vi "Init Async State Vars.vi"(8 "Error in":errorcluster, 10 "Async Parameters":T4) -> (0 "Error out":errorcluster, 3 "Async State Vars":T1)   [LabVIEW 2015, in "Waveform-Processing-Custom-Device Engine.lvlib"]
uses:
  Waveform-Processing-Custom-Device Engine.lvlib
  Types/Async Parameters.ctl
  Types/Async FIFOs.ctl
  <vilib>/NI Veristand/Custom Device API/Waveform Data Reference.ctl
  Types/Async State Vars.ctl
  <vilib>/NI Veristand/Custom Device Waveform API/Single Waveform Read (DBL)/Single Waveform Read (DBL).lvclass
  <vilib>/NI Veristand/Custom Device Waveform API/Single Waveform Write (DBL)/Single Waveform Write (DBL).lvclass
  <vilib>/NI VeriStand/Custom Device API/Custom Device API.lvlib
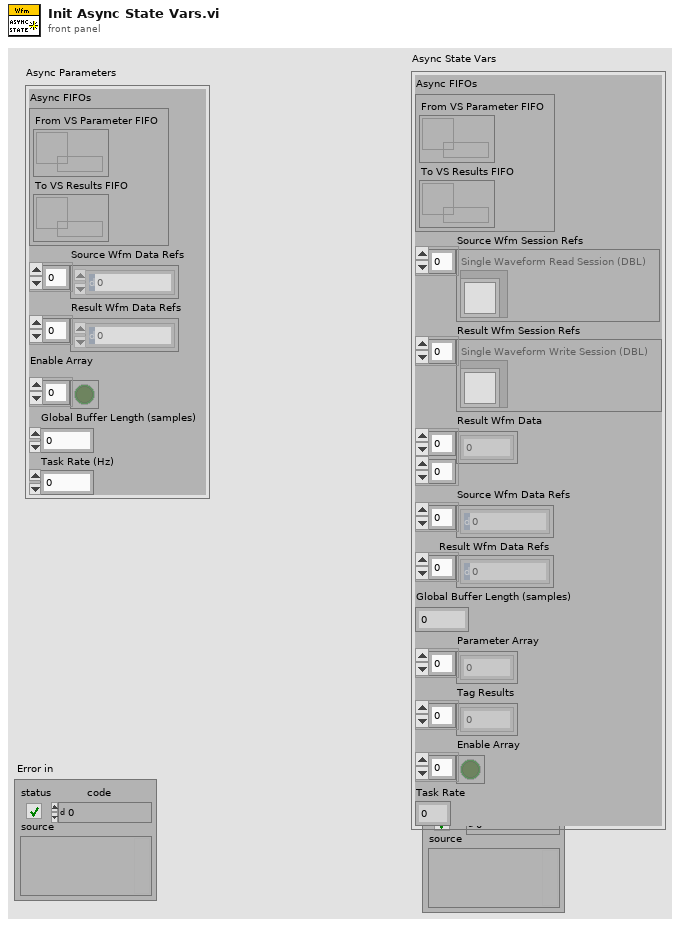
[diagram p1: front panel]
types:
  T1 = typedef "Waveform-Processing-Custom-Device Engine.lvlib/Async State Vars.ctl" = cluster{"Async FIFOs":T2, "Source Wfm Session Refs":refnum<class "Single Waveform Read (DBL).lvclass">[], "Result Wfm Session Refs":refnum<class "Single Waveform Write (DBL).lvclass">[], "Result Wfm Data":dbl[][], "Source Wfm Data Refs":T3[], "Result Wfm Data Refs":T3[], "Global Buffer Length (samples)":dbl, "Parameter Array":dbl[], "Tag Results":dbl[], "Enable Array":bool[], "Task Rate":dbl}
  T2 = typedef "Waveform-Processing-Custom-Device Engine.lvlib/Async FIFOs.ctl" = cluster{"From VS Parameter FIFO":refnum<k33>, "To VS Results FIFO":refnum<k33>}
  T3 = typedef "Custom Device API.lvlib/Waveform Data Reference.ctl" = i32
  T4 = typedef "Waveform-Processing-Custom-Device Engine.lvlib/Async Parameters.ctl" = cluster{"Async FIFOs":T2, "Source Wfm Data Refs":T3[], "Result Wfm Data Refs":T3[], "Enable Array":bool[], "Global Buffer Length (samples)":dbl, "Task Rate (Hz)":dbl}
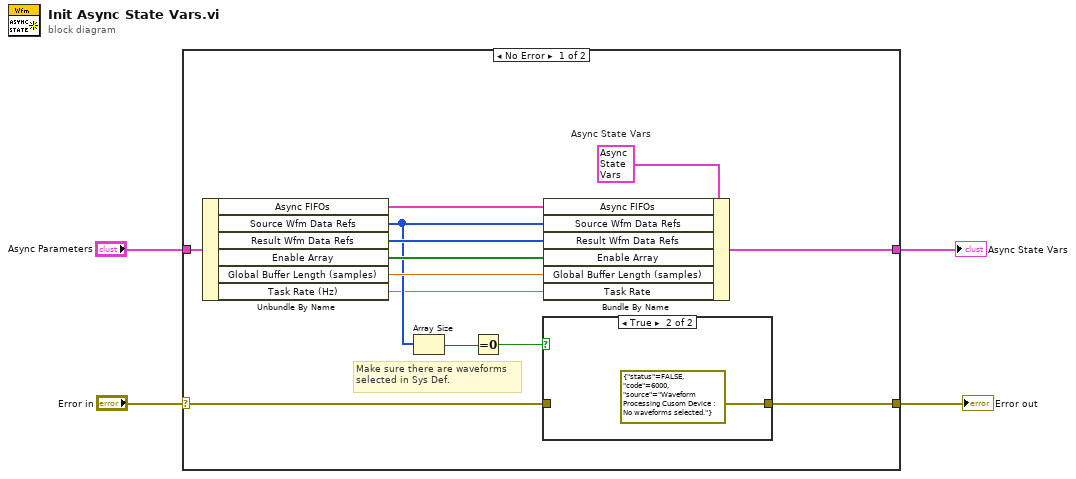
[diagram p0: block diagram]
diagram:
  n1 = case shown="No Error" "Error in" {
    selector: "Error in" -> [w7 w20]
    tunnel: [w6 w20] -> w3
    tunnel: "Async Parameters" -> [w17 _]
    tunnel: [w13 _] -> w1
    frame No Error {
      w16 = T1 {"Async FIFOs"={"From VS Parameter FIFO"=refnum, "To VS Results FIFO"=refnum}, "Source Wfm Session Refs"=[], "Result Wfm Session Refs"=[], "Result Wfm Data"=[], "Source Wfm Data Refs"=[], "Result Wfm Data Refs"=[], "Global Buffer Length (samples)"=0.0, "Parameter Array"=[], "Tag Results"=[], "Enable Array"=[], "Task Rate"=0.0}  # Async State Vars
      # "Make sure there are waveforms\nselected in Sys Def."
      n2 = Unbundle By Name(w17) -> ("Async FIFOs"=w15:T2, "Source Wfm Data Refs"=w10:T3[], "Result Wfm Data Refs"=w14:T3[], "Enable Array"=w12:bool[], "Global Buffer Length (samples)"=w11:dbl, "Task Rate (Hz)"=w5:dbl)
      n3 = Array Size(array=w10) -> (size(s)=w9:i32)
      n4 = Equal To 0?(x=w9) -> (x = 0?=w8:bool)
      n5 = case shown="True" w8 {
        tunnel: w7 -> [w18 _]
        tunnel: [w18 errorcluster {"status"=FALSE, "code"=6000, "source"="Waveform Processing Cusom Device : No waveforms selected."} ("error IO")] -> w6
        frame False {
        }
        frame True {
        }
      }
      n6 = Bundle By Name(cluster=w16, "Async FIFOs"=w15, "Source Wfm Data Refs"=w10, "Result Wfm Data Refs"=w14, "Enable Array"=w12, "Global Buffer Length (samples)"=w11, "Task Rate"=w5) -> (w13:T1)
    }
    frame Error {
    }
  }
  "Error out" <- w3
  "Async State Vars" <- w1
